vi "FRCts20_Backend_Dyn_Load_VIs.vi"(8 "error in":errorcluster, 11 "VI Names":path[](array[path])) -> (0 "error out":errorcluster, 3 "VI Names and Refnums":T1[](array[typedef]))   [LabVIEW 2014, in "FRCts20_Backend_Engine.lvlib"]
uses:
  FRCts20_Backend_Engine.lvlib
  FRCts20_Backend_Dyn_Refnums.ctl
  INI_Accessor/FRCts20_Backend_INI Controller.lvclass
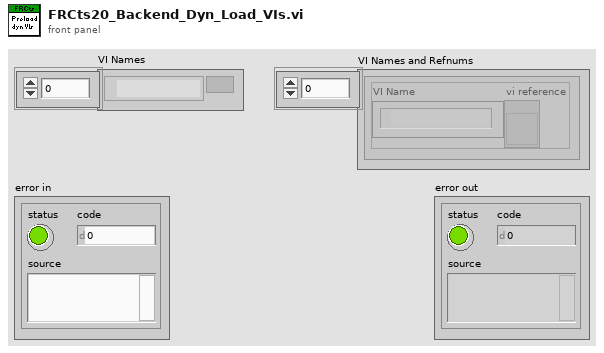
[diagram p1: front panel]
types:
  T1 = typedef "FRCts20_Backend_Engine.lvlib/FRCts20_Backend_Dyn_Refnums.ctl" = cluster{"VI Name":path, "vi reference":refnum<vi>}
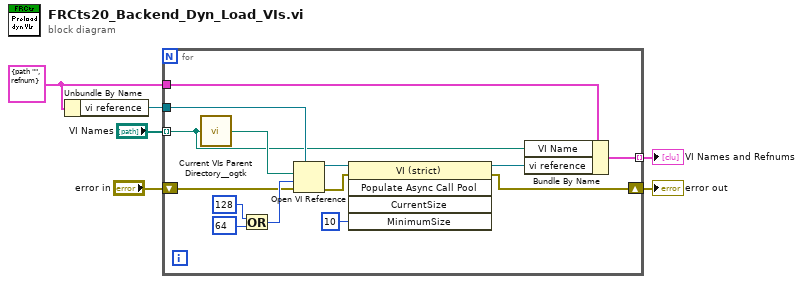
[diagram p0: block diagram]
diagram:
  w5 = T1 {"VI Name"=path "", "vi reference"=refnum} ("Dynamic VIs")
  n1 = Unbundle By Name(w5) -> ("vi reference"=w6:refnum<vi>)
  n2 = for {
    tunnel: "VI Names" -> [w8] mode=indexing
    tunnel: w6 -> [w16]
    tunnel: w5 -> [w12]
    shift-right: [w10] -> w2
    shift-left: "error in" -> [w9]
    tunnel: [w7] -> w1 mode=indexing
    n3 = call "Current VIs Parent Directory__ogtk.vi"("Relative path (.)"=w8) -> ("Parent Directory (+ Relative)"=w20:path)  [unwired: 4 in]
    n4 = Or(x=128, y=64) -> (x .or. y?=w17:i32)
    n5 = Open VI Reference(type specifier VI Refnum (for type only)=w16, vi path=w20, options=w17, error in (no error)=w9) -> (vi reference=w15:refnum<vi>, error out=w14:errorcluster)  [unwired: 2 in]
    n6 = invoke class="VI (strict)" method="Populate Async Call Pool"(reference=w15, error in=w14, "MinimumSize"=10 ("Minimum Size")) -> (reference out=w11:refnum<vi>, error out=w10:errorcluster)  [unwired: 2 in, 3 out]
    n7 = Bundle By Name(cluster=w12, "VI Name"=w8, "vi reference"=w11) -> (w7:T1)
  }
  "error out" <- w2
  "VI Names and Refnums" <- w1
